vi "advanced gyro encoder safety.vi"(0 "Input":dbl, 5 "Configuration":T2={"Min Rate"=0.0, "Cutoff Rate"=0.2, "Reverse Limit"=0.0, "Forward Limit"=0.0}, 6 "Encoder Rate":dbl, 8 "Encoder Distance":dbl, 10 "Gyro Angular Rate":dbl) -> (14 "Output":dbl, 19 "Safety Errors":T1)   [LabVIEW 2014]
panel:
  # "A Super Safe VI"
  # "Sensor Input"
  # "Safety Errors"
  # "Desired Input"
  # "Configuration"
  # "Resulting Safe Output"
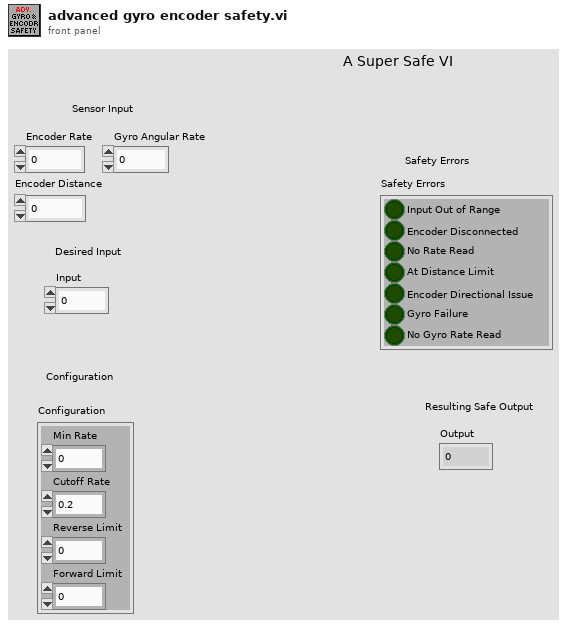
[diagram p1: front panel]
types:
  T1 = cluster{"Input Out of Range":bool, "At Distance Limit":bool, "Encoder Directional Issue":bool, "No Rate Read":bool, "Encoder Disconnected":bool, "Gyro Failure":bool, "No Gyro Rate Read":bool}
  T2 = cluster{"Min Rate":dbl, "Cutoff Rate":dbl, "Reverse Limit":dbl, "Forward Limit":dbl}
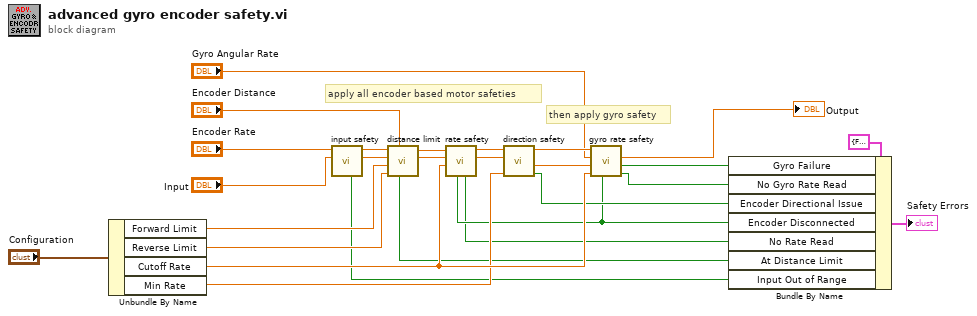
[diagram p0: block diagram]
diagram:
  # "then apply gyro safety"
  # "apply all encoder based motor safeties"
  n1 = Unbundle By Name("Configuration") -> ("Forward Limit"=w13:dbl, "Reverse Limit"=w12:dbl, "Cutoff Rate"=w11:dbl, "Min Rate"=w10:dbl)
  n2 = call "input safety.vi"("Desired Rate"="Input", "Encoder Rate"="Encoder Rate") -> ("Safe Rate"=w27:dbl, "Encoder Rate Out"=w26:dbl, "Input Out of Range"=w2:bool)  [unwired: 7 in]
  n3 = call "distance limit.vi"("Encoder Rate"=w26, "Encoder Distance"="Encoder Distance", "Desired Rate"=w27, "Forward Limit"=w13, "Reverse Limit"=w12) -> ("At Distance Limit"=w3:bool, "Encoder Rate Out"=w23:dbl, "Output Rate"=w25:dbl)  [unwired: 1 in]
  n4 = call "rate safety.vi"("Cutoff Rate"=w11, "Desired Rate"=w25, "Encoder Rate"=w23) -> ("Output Rate"=w24:dbl, "Encoder Rate Out"=w18:dbl, "No Rate Read"=w4:bool, "Encoder Failure"=w5:bool)  [unwired: 5 in]
  n5 = call "direction safety.vi"("Min Rate"=w10, "Desired Rate"=w24, "Encoder Rate"=w18) -> ("Encoder Directional Issue"=w6:bool, "Super Safe Rate"=w19:dbl, "Encoder Rate Out"=w17:dbl)  [unwired: 2 in]
  n6 = call "gyro rate safety.vi"("Encoder Failure"=w5, "Cutoff Rate"=w11, "Input"=w19, "Gyro Angular Rate"="Gyro Angular Rate", "Encoder Rate"=w17) -> ("No Gyro Rate Read"=w7:bool, "Gyro Failure"=w8:bool, "Output"=→"Output":dbl)  [unwired: 3 in, 1 out]
  n7 = Bundle By Name(cluster=T1 {"Input Out of Range"=FALSE, "At Distance Limit"=FALSE, "Encoder Directional Issue"=FALSE, "No Rate Read"=FALSE, "Encoder Disconnected"=FALSE, "Gyro Failure"=FALSE, "No Gyro Rate Read"=FALSE} ("Safety Errors"), "Gyro Failure"=w8, "No Gyro Rate Read"=w7, "Encoder Directional Issue"=w6, "Encoder Disconnected"=w5, "No Rate Read"=w4, "At Distance Limit"=w3, "Input Out of Range"=w2) -> (→"Safety Errors":T1)
